vi "Loop Timeout.vi"(1 "App in":refnum<class "App.lvclass">) -> (0 "Timeout":i32)   [LabVIEW 2020, in "AR Example.lvlib" / "App.lvclass"]
uses:
  App.lvclass
  App.lvclass/App.ctl
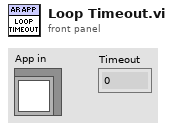
[diagram p1: front panel]
types:
  T1 = typedef "AR Example.lvlib/App.lvclass/Timeout Action.ctl" = enum16{"None", "Capture Preview Image"}
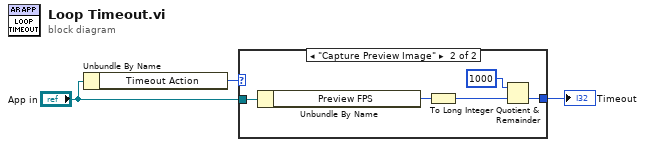
[diagram p0: block diagram]
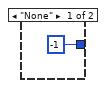
[diagram p2: hidden frame]
diagram:
  n1 = Unbundle By Name("App in") -> ("Timeout Action"=w3:T1)
  n2 = case shown="\"Capture Preview Image\"" w3 {
    tunnel: [-1 w5] -> w2
    tunnel: "App in" -> [_ w9]
    frame "None" {
    }
    frame "Capture Preview Image" {
      n3 = Unbundle By Name(w9) -> ("Preview FPS"=w7:u8)
      n4 = To Long Integer(number=w7) -> (32bit integer=w6:i32)
      n5 = Quotient & Remainder(x=1000, y=w6) -> (floor(x/y)=w5:i32)  [unwired: 1 out]
    }
  }
  "Timeout" <- w2
